vi "Start.vi"(4 "init":bool, 5 "ptr":i64, 6 "batchSize":u32=50, 7 "error in (no error)":errorcluster) -> (0 "wrongLayer":u32, 1 "ptr out":i64, 2 "Layers":u32, 3 "error out":errorcluster)   [LabVIEW 2016, in "CNet.lvlib"]
uses:
  CNet.lvlib
  Users/jg754/Documents/Visual Studio 2015/Projects/CLearn/x64/Release/CLearn.dll
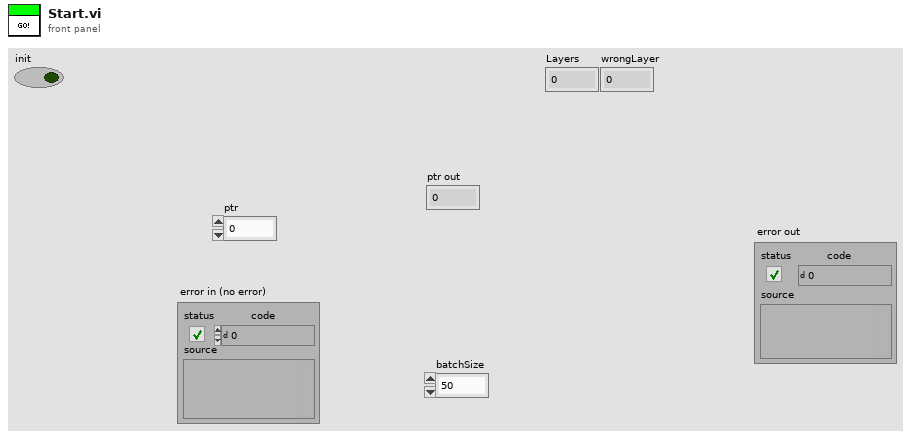
[diagram p1: front panel]
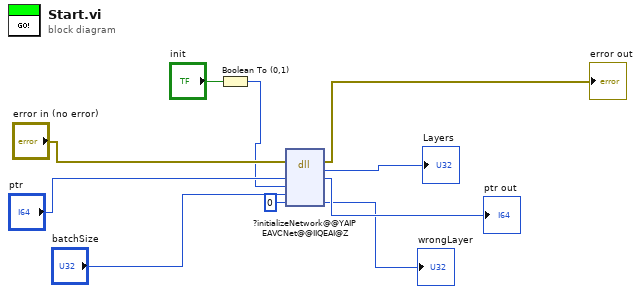
[diagram p0: block diagram]
diagram:
  n1 = Boolean To (0,1)(Boolean="init") -> (0, 1=w3:i16)
  n2 = dll-call lib="C:/Users/jg754/Documents/Visual Studio 2015/Projects/CLearn/x64/Release/CLearn.dll" fn="?initializeNetwork@@YAIPEAVCNet@@IIQEAI@Z"(error in="error in (no error)", "ptr"="ptr", "init"=w3, "batchSize"="batchSize", "wrongLayer"=u32 0) -> (error out=→"error out":errorcluster, "return"=→"Layers":u32, "ptr"=→"ptr out":i64, "wrongLayer"=→"wrongLayer":u32)  [unwired: 4 in, 1 out]
